vi "DCPower_TurnOff_byIndividualChannel_KeepReference.vi"(2 "error in (no error)":errorcluster, 3 "DCPower_ToggleIndex":i32[](array[numeric]), 4 "DCPower_byChannel in":T1(array[cluster])) -> (0 "error out":errorcluster, 1 "DCPower_byChannel out":T1(array[cluster]))   [LabVIEW 2019]
panel:
  in  "DCPower_byChannel in 2":T1(array[cluster])
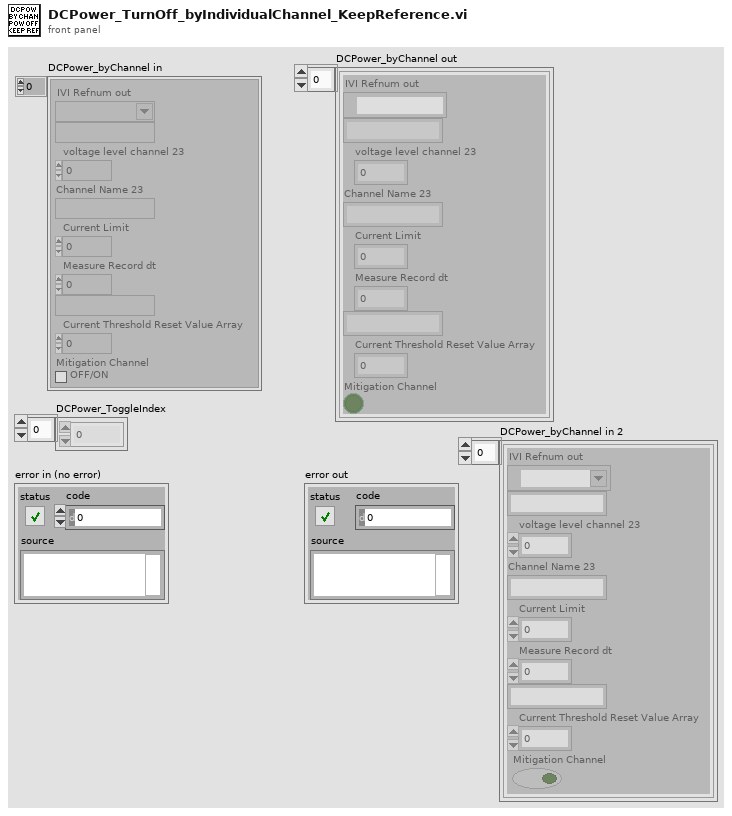
[diagram p1: front panel]
types:
  T1 = cluster{"IVI Refnum out":refnum<k15>, string, "voltage level channel 23":dbl, "Channel Name 23":string, "Current Limit":dbl, "Measure Record dt":dbl, string, "Current Threshold Reset Value Array":dbl, "Mitigation Channel":bool}[]
  T2 = cluster{"IVI Refnum out":refnum<k15>, string, "voltage level channel 23":dbl, "Channel Name 23":string, "Current Limit":dbl, "Measure Record dt":dbl, string, "Current Threshold Reset Value Array":dbl, "Mitigation Channel":bool}
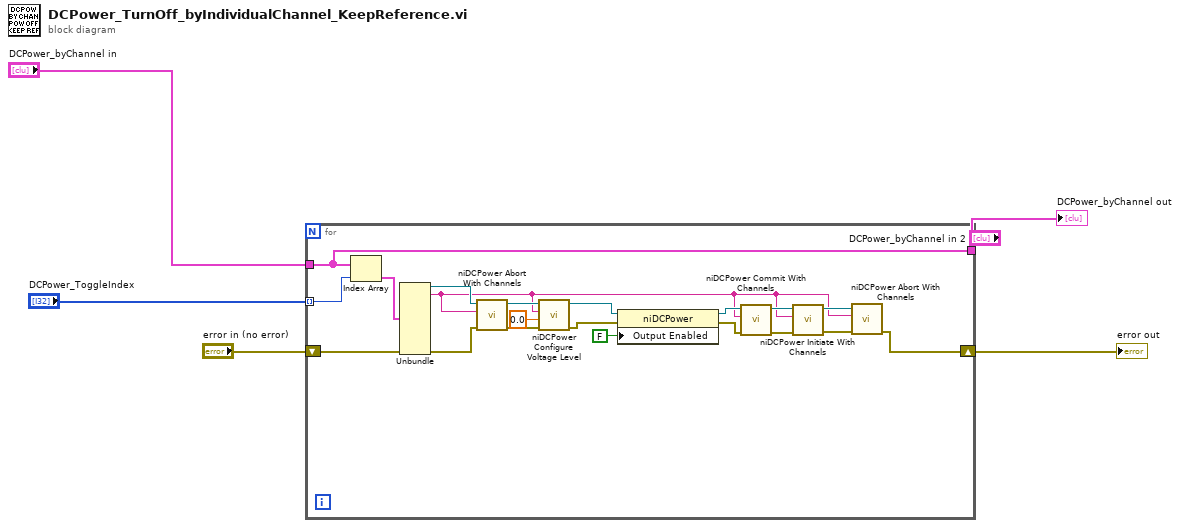
[diagram p0: block diagram]
diagram:
  n1 = for {
    tunnel: "DCPower_byChannel in" -> [w6]
    tunnel: "DCPower_ToggleIndex" -> [w24] mode=indexing
    shift-right: [w7] -> w4
    shift-left: "error in (no error)" -> [w21]
    tunnel: [w6] -> w1
    n2 = Index Array(array=w6, index=w24) -> (element=w23:T2)
    n3 = Unbundle(w23) -> ("IVI Refnum out"=w22:refnum<k15>, w8:string)  [unwired: 7 out]
    n4 = call <instrlib>:"niDCPower Abort With Channels.vi"("error in (no error)"=w21, "channel name"=w8, "instrument handle"=w22) -> ("error out"=w20:errorcluster, "instrument handle out"=w19:refnum<k15>)  [unwired: 7 in]
    n5 = call <instrlib>:"niDCPower Configure Voltage Level.vi"("error in (no error)"=w20, "voltage level"=0.0, "channel name"=w8, "instrument handle"=w19) -> ("error out"=w16:errorcluster, "instrument handle out"=w17:refnum<k15>)  [unwired: 6 in]
    n6 = property class="niDCPower"(reference=w17, error in=w16, "Output Enabled"=FALSE ("Source:Output Enabled")) -> (reference out=w13:refnum<k15>, error out=w14:errorcluster)
    n7 = call <instrlib>:"niDCPower Commit With Channels.vi"("error in (no error)"=w14, "channel name"=w8, "instrument handle"=w13) -> ("error out"=w12:errorcluster, "instrument handle out"=w11:refnum<k15>)  [unwired: 7 in]
    n8 = call <instrlib>:"niDCPower Initiate With Channels.vi"("error in (no error)"=w12, "channel name"=w8, "instrument handle"=w11) -> ("error out"=w10:errorcluster, "instrument handle out"=w9:refnum<k15>)  [unwired: 7 in]
    n9 = call <instrlib>:"niDCPower Abort With Channels.vi"("error in (no error)"=w10, "channel name"=w8, "instrument handle"=w9) -> ("error out"=w7:errorcluster)  [unwired: 7 in, 1 out]
  }
  "error out" <- w4
  "DCPower_byChannel out" <- w1
